vi "Print Console.vi"() -> ()   [LabVIEW 2010]
doc: "이 인쇄 큐 콘솔은 인쇄 작업 제출의 컨트롤을 시뮬레이션하고 처리 중인 인쇄 작업의 상태를 모니터합니다."
uses:
  Print Indicators.ctl
  Print Processing States.ctl
panel:
  out "인쇄 인디케이터":T1={"대기 중"=TRUE, "초기화 중"=FALSE, "인쇄 중"=FALSE, "작업 개수"=0}
  out "큐 인쇄 작업":i32(slide) scale=0.0..25.0
  in  "큐 이벤트":bool
  in  "정지":bool
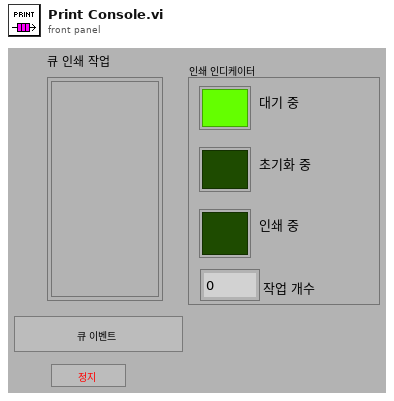
[diagram p1: front panel]
types:
  T1 = typedef "Print Indicators.ctl" = cluster{"대기 중":bool, "초기화 중":bool, "인쇄 중":bool, "작업 개수":i32}
  T2 = typedef "Print Processing States.ctl" = enum16{"대기", "셋업 초기화", "셋업", "인쇄 초기화", "인쇄", "종료"}
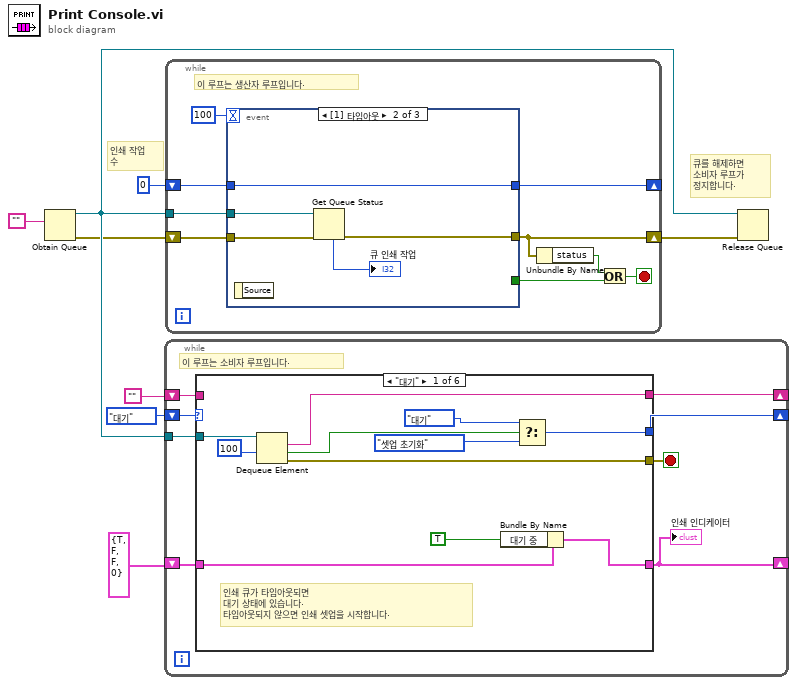
[diagram p0: block diagram]
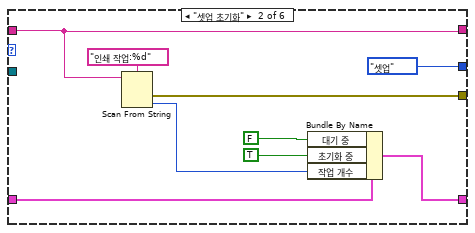
[diagram p2: hidden frame]
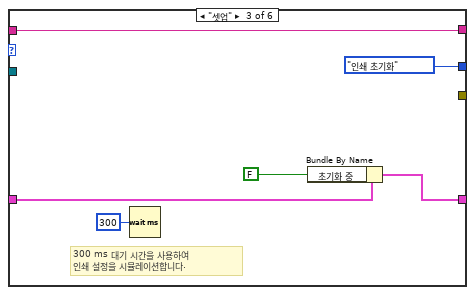
[diagram p3: hidden frame]
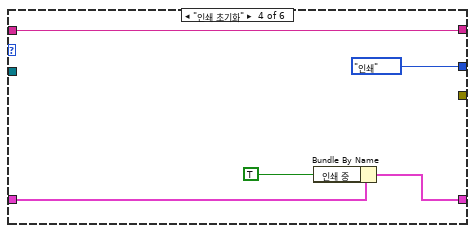
[diagram p4: hidden frame]
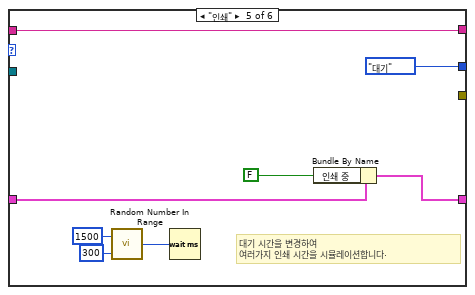
[diagram p5: hidden frame]
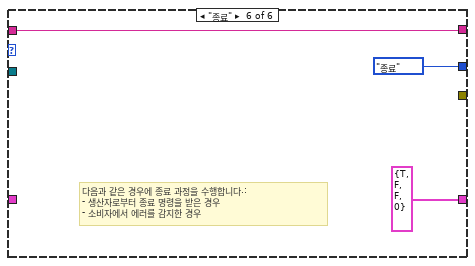
[diagram p6: hidden frame]
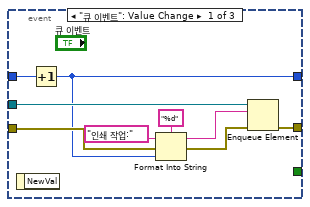
[diagram p7: hidden frame]
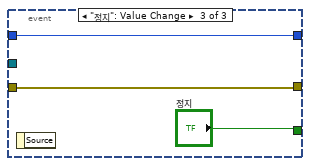
[diagram p8: hidden frame]
diagram:
  # "인쇄 작업\n수"
  # "큐를 해제하면\n소비자 루프가\n정지합니다."
  n1 = Obtain Queue ("큐 얻기")(element data type="") -> (queue out=w7:refnum<queue>, error out=w1:errorcluster)  [unwired: 4 in, 1 out]
  n2 = while "While 루프" {
    tunnel: w7 -> [w16]
    shift-right: [w10] -> _
    shift-left: Print_Processing_States."대기" ("Enum") -> [w15]
    shift-right: [w13] -> _
    shift-left: T1 {"대기 중"=TRUE, "초기화 중"=FALSE, "인쇄 중"=FALSE, "작업 개수"=0} ("Print LEDs") -> [w14]
    shift-right: [w11] -> _
    shift-left: "" -> [w12]
    stop <- w9 stop-if-true
    # "이 루프는 소비자 루프입니다."
    n3 = case "케이스 구조" shown="\"대기\"" w15 {
      tunnel: w16 -> [w27 _ _ _ _ _]
      tunnel: [w26 w28 _ _ _ _] -> w9
      tunnel: w14 -> [w21 w35 w41 w46 w54 _]
      tunnel: [w20 w34 w40 w45 w53 T1 {"대기 중"=TRUE, "초기화 중"=FALSE, "인쇄 중"=FALSE, "작업 개수"=0} ("Print LEDs")] -> w13
      tunnel: [w18 Print_Processing_States."셋업" ("Enum") Print_Processing_States."인쇄 초기화" ("Enum") Print_Processing_States."인쇄" ("Enum") Print_Processing_States."대기" ("Enum") Print_Processing_States."종료" ("Enum")] -> w10
      tunnel: [w17 w31 w37 w43 w48 w56] -> w11
      tunnel: w12 -> [_ w31 w37 w43 w48 w56]
      frame "대기" {
        # "인쇄 큐가 타임아웃되면\n대기 상태에 있습니다.\n타임아웃되지 않으면 인쇄 셋업을 시작합니다."
        n4 = Dequeue Element(queue=w27, timeout in ms (-1)=100) -> (element=w17:string, timed out?=w19:bool, error out=w26:errorcluster)  [unwired: 1 in, 1 out]
        n5 = Bundle By Name(cluster=w21, "대기 중"=TRUE ("Waiting for\nnew job...")) -> (w20:T1)
        n6 = Select(t=Print_Processing_States."대기" ("Enum"), s=w19, f=Print_Processing_States."셋업 초기화" ("Enum")) -> (s? t:f=w18:T2)
      }
      frame "셋업 초기화" {
        n7 = Scan From String(format string="인쇄 작업:%d", input string=w31) -> (error out=w28:errorcluster, output 1=w29:i32)  [unwired: 3 in, 2 out]
        n8 = Bundle By Name(cluster=w35, "대기 중"=FALSE ("Waiting for\nnew job..."), "초기화 중"=TRUE ("Waiting for\nnew job..."), "작업 개수"=w29) -> (w34:T1)
      }
      frame "셋업" {
        # "300 ms 대기 시간을 사용하여\n인쇄 설정을 시뮬레이션합니다."
        n9 = Wait (ms)(milliseconds to wait=u32 300) -> ()  [unwired: 1 out]
        n10 = Bundle By Name(cluster=w41, "초기화 중"=FALSE ("Waiting for\nnew job...")) -> (w40:T1)
      }
      frame "인쇄 초기화" {
        n11 = Bundle By Name(cluster=w46, "인쇄 중"=TRUE ("Waiting for\nnew job...")) -> (w45:T1)
      }
      frame "인쇄" {
        # "대기 시간을 변경하여\n여러가지 인쇄 시간을 시뮬레이션합니다."
        n12 = call "Random Number In Range.vi"("하위 리미트"=u32 300 ("Lower Limit"), "상위 리미트"=u32 1500 ("Upper Limit")) -> ("임의의 수"=w49:u32)
        n13 = Wait (ms)(milliseconds to wait=w49) -> ()  [unwired: 1 out]
        n14 = Bundle By Name(cluster=w54, "인쇄 중"=FALSE ("Waiting for\nnew job...")) -> (w53:T1)
      }
      frame "종료" {
        # "다음과 같은 경우에 종료 과정을 수행합니다.:\n- 생산자로부터 종료 명령을 받은 경우\n- 소비자에서 에러를 감지한 경우"
      }
    }
    "인쇄 인디케이터" <- w13
  }
  n15 = while "While 루프" {
    tunnel: w7 -> [w67]
    shift-right: [w61] -> _
    shift-left: 0 -> [w62]
    shift-right: [w60] -> w2
    shift-left: w1 -> [w59]
    stop <- w65 stop-if-true
    # "이 루프는 생산자 루프입니다."
    n16 = event "이벤트 구조" shown="[1] 타임아웃" {
      selector: _ -> [_ _ _]
      dyn-events: _ -> [_ _ _]
      timeout: 100 -> [_ _ _]
      tunnel: w67 -> [w76 w79 _]
      tunnel: w59 -> [w74 w80 w82]
      tunnel: [w75 w78 w82] -> w60
      tunnel: [_ _ "정지"] -> w66
      tunnel: w62 -> [w70 w77 w83]
      tunnel: [w68 w77 w83] -> w61
      event "큐 이벤트": Value Change {
        n17 = event-data() -> ()  [unwired: 1 in, 1 out]
        n18 = Increment(x=w70) -> (x+1=w68:i32)
        n19 = Format Into String(format string="%d", initial string="인쇄 작업:", error in=w74, w68) -> (resulting string=w69:string, error out=w73:errorcluster)
        n20 = Enqueue Element(queue=w76, element=w69, error in (no error)=w73) -> (error out=w75:errorcluster)  [unwired: 1 in, 2 out]
      }
      event Timeout {
        n21 = event-data() -> ()  [unwired: 1 in, 1 out]
        n22 = Get Queue Status(queue=w79, error in (no error)=w80) -> (error out=w78:errorcluster, # elements in queue=→"큐 인쇄 작업":i32)  [unwired: 1 in, 6 out]
      }
      event "정지": Value Change {
        n23 = event-data() -> ()  [unwired: 1 in, 1 out]
      }
    }
    n24 = Unbundle By Name ("이름으로 풀기")(w60) -> ("status"=w64:bool)
    n25 = Or(x=w64, y=w66) -> (x .or. y?=w65:bool)
  }
  n26 = Release Queue ("큐 해제")(queue=w7, error in (no error)=w2) -> ()  [unwired: 1 in, 3 out]
